vi "Cluster write one.vi"(9 "new element/subarray":bool, 10 "index of cluster":i32, 11 "WT1600.lvlib:WT1600.lvclass":refnum<class "WT1600.lvclass">) -> (3 "WT1600 out":refnum<class "WT1600.lvclass">)   [LabVIEW 2012, in "WT1600.lvlib" / "WT1600.lvclass"]
uses:
  WT1600.lvclass
  WT1600.lvclass/WT1600.ctl
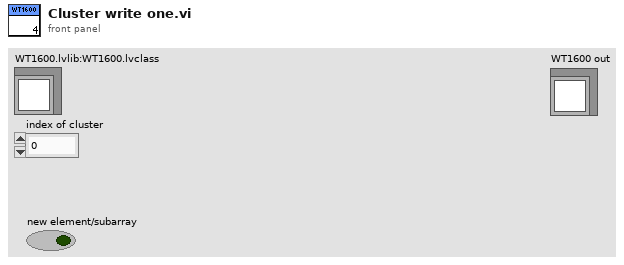
[diagram p1: front panel]
types:
  T1 = cluster{"Card 1":bool, "Card 2":bool, "Card 3":bool, "Card 4":bool, "Card 5":bool, "Card 6":bool}
  T2 = cluster{"Value[0]":bool, "Value[1]":bool, "Value[2]":bool, "Value[3]":bool, "Value[4]":bool, "Value[5]":bool}
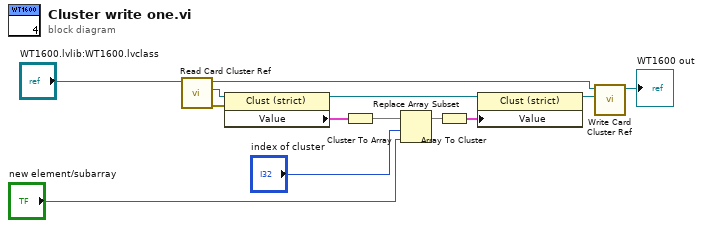
[diagram p0: block diagram]
diagram:
  n1 = call "Read Card Cluster Ref.vi"("WT1600 in"="WT1600.lvlib:WT1600.lvclass") -> ("error out"=w12:errorcluster, "Card Cluster Ref"=w2:refnum<vi>, "WT1600 out"=w4:refnum<class "WT1600.lvclass">)  [unwired: 8 in]
  n2 = property class="Clust (strict)"(reference=w2, error in=w12) -> (reference out=w1:refnum<vi>, "Value"=w11:T1)  [unwired: 1 out]
  n3 = Cluster To Array(cluster=w11) -> (array=w10:bool[])
  n4 = Replace Array Subset(array=w10, new element="new element/subarray", index="index of cluster") -> (w7:bool[])
  n5 = Array To Cluster(array=w7) -> (cluster=w6:T2)
  n6 = property class="Clust (strict)"(reference=w1, "Value"=w6) -> (reference out=w5:refnum<vi>)  [unwired: 1 in, 1 out]
  n7 = call "Write Card Cluster Ref.vi"("Card Cluster Ref"=w5, "WT1600 in"=w4) -> ("WT1600 out"=→"WT1600 out":refnum<class "WT1600.lvclass">)  [unwired: 8 in, 1 out]
